vi "calc_RH_subVI.vi"(6 "both flows off?":bool, 9 "vapor flow":dbl, 10 "gas flow":dbl, 11 "low pressure":dbl) -> (1 "RH":string)   [LabVIEW 2014]
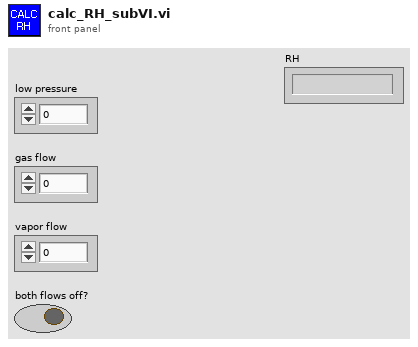
[diagram p1: front panel]
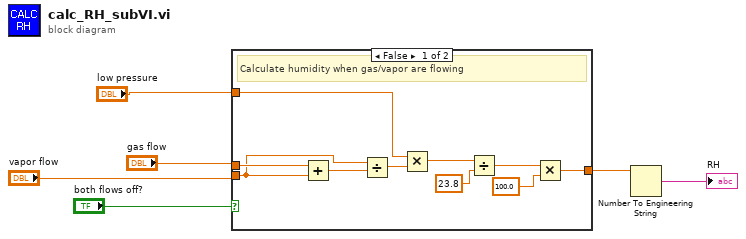
[diagram p0: block diagram]
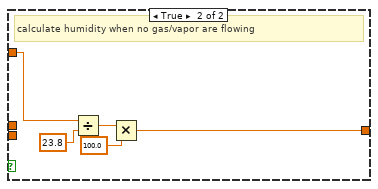
[diagram p2: hidden frame]
diagram:
  n1 = case shown="False" "both flows off?" {
    tunnel: "low pressure" -> [w8 w18]
    tunnel: [w7 w17] -> w2
    tunnel: "gas flow" -> [w16 _]
    tunnel: "vapor flow" -> [w14 _]
    frame False {
      # "Calculate humidity when gas/vapor are flowing"
      n2 = Add(x=w16, y=w14) -> (x+y=w15:dbl)
      n3 = Divide(x=w14, y=w15) -> (x/y=w9:dbl)
      n4 = Multiply(x=w8, y=w9) -> (x*y=w10:dbl)
      n5 = Divide(x=w10, y=23.8) -> (x/y=w12:dbl)
      n6 = Multiply(x=w12, y=100.0) -> (x*y=w7:dbl)
    }
    frame True {
      # "calculate humidity when no gas/vapor are flowing"
      n7 = Divide(x=w18, y=23.8) -> (x/y=w20:dbl)
      n8 = Multiply(x=w20, y=100.0) -> (x*y=w17:dbl)
    }
  }
  n9 = Number To Engineering String(4:w2) -> (0:→"RH":string)  [unwired: 3 in]
